vi "Actor Core.vi"(8 "error in":errorcluster, 11 "State in":refnum<class "Forward Drive.lvclass">) -> (0 "error out":errorcluster, 3 "Actor out":refnum<class "Actor.lvclass">)   [LabVIEW 2014, in "Forward Drive.lvlib" / "Forward Drive.lvclass"]
doc: "(<B>Filename</B>: Actor Framework.lvlib:Actor.lvclass:Actor Core.vi)\n\nThis override invokes Entry.vi on the initial state, prior to calling the parent Actor Core. Adding this behavior to Actor Core (instead of an override of Pre Launch Init.vi) allows the initial state to launch a nested actor as part of its entry behavior.\n\nReceives messages to the actor, reacts to them, and initiates any error handling that may shut the actor down.\n\nDescendant classes may override this VI to append parallel tasks for the actor to complete while it handles messages. Overrides use the Call Parent Method node."
uses:
  Forward Drive.lvclass
  <vilib>/ActorFramework/Actor/Actor.lvclass
  Virtual Robot/Virtual Forward Drive/Virtual Forward Drive Class/Forward Drive State.ctl
  Forward Drive.lvclass/Forward Drive.ctl
  Motor with Encoders/Motors with Encoders Class/Motors with Encoders.lvclass
  Robot Actor Framework/System Actor/System Actor Class/System Actor.lvclass
panel:
  in  "Forward Drive  State":T1 {"Right Drive Power" min=-1.0 max=1.0 scale=-1.0..1.0; "Left Drive Power" min=-1.0 max=1.0 scale=-1.0..1.0}
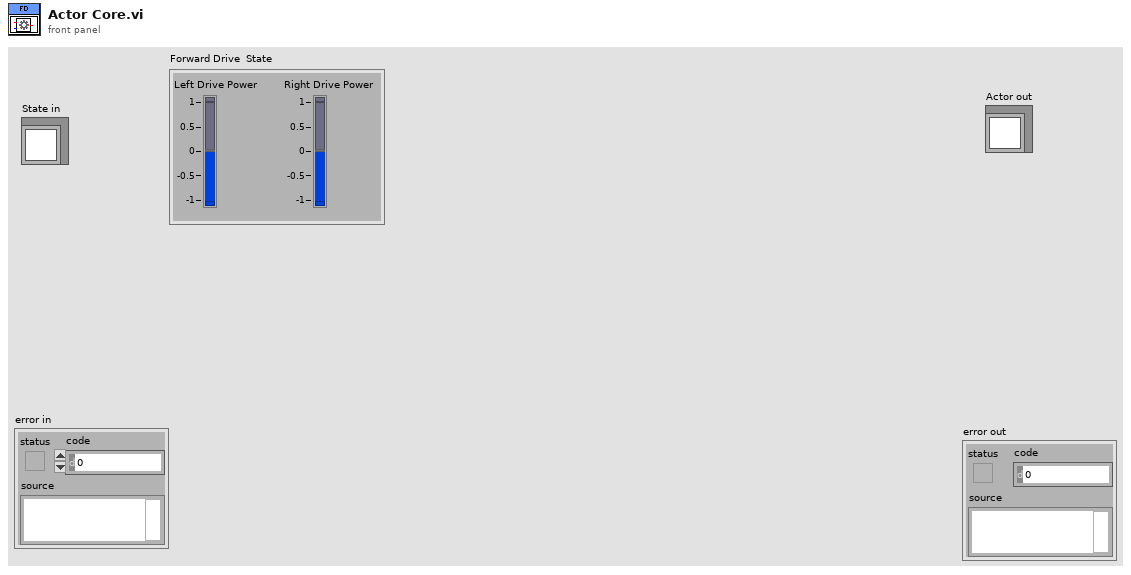
[diagram p1: front panel]
types:
  T1 = typedef "Forward Drive.lvlib/Forward Drive.lvclass/Forward Drive State.ctl" = cluster{"Left Drive Power":dbl, "Right Drive Power ":dbl}
  T2 = typedef "Motors with Encoders.lvlib/Motors with Encoders.lvclass/Motors with Encoders Config.ctl" = cluster{"Counts  Per Revolution":u32, "Invert Encoder Direction":bool, "Diameter of Revolution":dbl, "Max RPM":dbl, "Encoder Control":bool}
  T3 = enum16{"Critical", "Error", "Warning", "Informational", "Debug"}
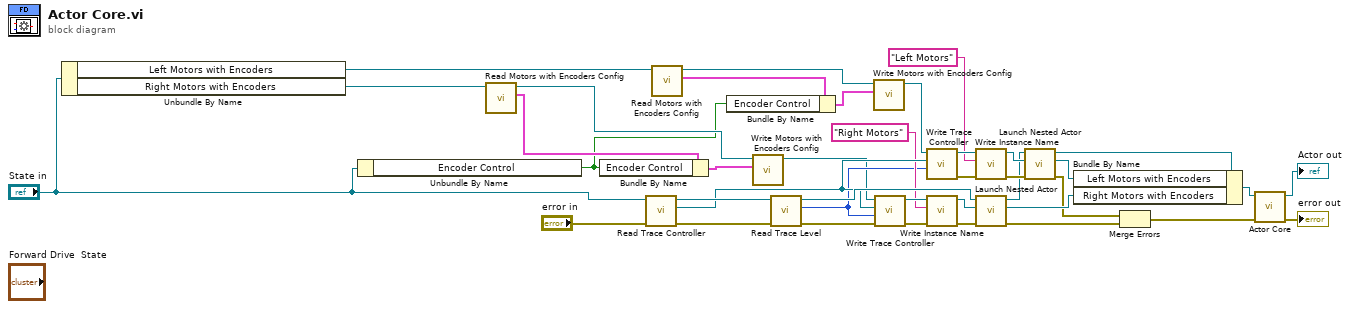
[diagram p0: block diagram]
diagram:
  n1 = Unbundle By Name("State in") -> ("Left Motors with Encoders"=w12:refnum<class "Motors with Encoders.lvclass">, "Right Motors with Encoders"=w8:refnum<class "Motors with Encoders.lvclass">)
  n2 = Unbundle By Name("State in") -> ("Encoder Control"=w1:bool)
  n3 = call-dynamic "Read Motors with Encoders Config.vi"("Motors with Encoders in"=w8) -> ("Config"=w5:T2, "Motors with Encoders out"=w7:refnum<class "Motors with Encoders.lvclass">)  [unwired: 8 in, 1 out]
  n4 = Bundle By Name(cluster=w5, "Encoder Control"=w1) -> (w2:T2)
  n5 = call-dynamic "Read Trace Controller.vi"("error in (no error)"="error in", "System Actor in"="State in") -> ("error out"=w30:errorcluster, "Trace Controller"=w32:refnum<class "Message Enqueuer.lvclass">, "System Actor out"=w33:refnum<class "Forward Drive.lvclass">)  [unwired: 7 in]
  n6 = call-dynamic "Read Motors with Encoders Config.vi"("Motors with Encoders in"=w12) -> ("Config"=w9:T2, "Motors with Encoders out"=w11:refnum<class "Motors with Encoders.lvclass">)  [unwired: 8 in, 1 out]
  n7 = Bundle By Name(cluster=w9, "Encoder Control"=w1) -> (w3:T2)
  n8 = call-dynamic "Write Motors with Encoders Config.vi"("Motors with Encoders Config"=w2, "Motors with Encoders in"=w7) -> ("Motors with Encoders out"=w6:refnum<class "Motors with Encoders.lvclass">)  [unwired: 8 in, 1 out]
  n9 = call-dynamic "Read Trace Level.vi"("error in (no error)"=w30, "System Actor in"=w33) -> ("error out"=w16:errorcluster, "Trace Level"=w17:T3, "System Actor out"=w35:refnum<class "Forward Drive.lvclass">)  [unwired: 7 in]
  n10 = call-dynamic "Write Motors with Encoders Config.vi"("Motors with Encoders Config"=w3, "Motors with Encoders in"=w11) -> ("Motors with Encoders out"=w10:refnum<class "Motors with Encoders.lvclass">)  [unwired: 8 in, 1 out]
  n11 = call-dynamic "Write Trace Controller.vi"("error in (no error)"=w16, "Trace Level"=w17, "Trace Controller"=w32, "System Actor in"=w6) -> ("error out"=w19:errorcluster, "System Actor out"=w25:refnum<class "Motors with Encoders.lvclass">)  [unwired: 6 in]
  n12 = call-dynamic "Write Trace Controller.vi"("Trace Level"=w17, "Trace Controller"=w32, "System Actor in"=w10) -> ("error out"=w21:errorcluster, "System Actor out"=w26:refnum<class "Motors with Encoders.lvclass">)  [unwired: 7 in]
  n13 = call-dynamic "Write Instance Name.vi"("error in (no error)"=w19, "Instance Name"="Right Motors", "System Actor in"=w25) -> ("error out"=w18:errorcluster, "System Actor out"=w24:refnum<class "Motors with Encoders.lvclass">)  [unwired: 7 in]
  n14 = call-dynamic "Write Instance Name.vi"("error in (no error)"=w21, "Instance Name"="Left Motors", "System Actor in"=w26) -> ("error out"=w20:errorcluster, "System Actor out"=w15:refnum<class "Motors with Encoders.lvclass">)  [unwired: 7 in]
  n15 = call <vilib>:"Launch Nested Actor.vi"("error in (no error)"=w18, "Nested Actor"=w24, "Caller Actor in"=w35) -> ("error out"=w28:errorcluster, "Nested Actor's Enqueuer"=w34:refnum<class "Message Enqueuer.lvclass">, "Caller Actor out"=w14:refnum<class "Forward Drive.lvclass">)  [unwired: 6 in]
  n16 = call <vilib>:"Launch Nested Actor.vi"("error in (no error)"=w20, "Nested Actor"=w15, "Caller Actor in"=w14) -> ("error out"=w27:errorcluster, "Nested Actor's Enqueuer"=w36:refnum<class "Message Enqueuer.lvclass">, "Caller Actor out"=w13:refnum<class "Forward Drive.lvclass">)  [unwired: 6 in]
  n17 = Bundle By Name(cluster=w13, "Left Motors with Encoders"=w36, "Right Motors with Encoders"=w34) -> (w37:refnum<class "Forward Drive.lvclass">)
  n18 = Merge Errors(w27, w28) -> (w29:errorcluster)
  n19 = call-parent "Actor Core.vi"("error in"=w29, "State in"=w37) -> ("error out"=→"error out":errorcluster, "Actor out"=→"Actor out":refnum<class "Actor.lvclass">)  [unwired: 8 in]
